vi "Check Next Step.vi"(8 "error in (no error)":errorcluster, 10 "Current Time":timestamp, 11 "Output Sequencer in":refnum<class "Output Sequencer.lvclass">) -> (0 "error out":errorcluster, 2 "Go to Next Step":bool, 3 "Output Sequencer out":refnum<class "Output Sequencer.lvclass">, 4 "Current Step End Timestamp":dbl)   [LabVIEW 2020, in "Output Sequencer.lvlib" / "Output Sequencer.lvclass"]
uses:
  Output Sequencer.lvclass
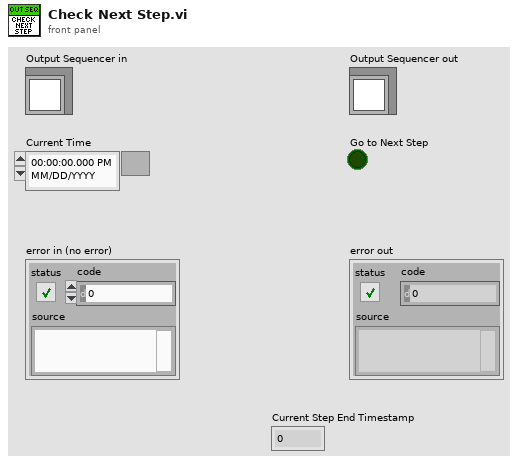
[diagram p1: front panel]
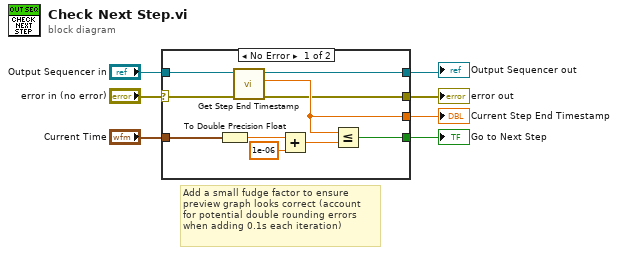
[diagram p0: block diagram]
diagram:
  # "Add a small fudge factor to ensure\npreview graph looks correct (account\nfor potential double rounding errors\nwhen adding 0.1s each iteration)"
  n1 = case shown="No Error" "error in (no error)" {
    selector: "error in (no error)" -> [w8 w18]
    tunnel: "Output Sequencer in" -> [w17 w19]
    tunnel: [w16 _] -> w6
    tunnel: [w15 _] -> w5
    tunnel: [w14 w18] -> w4
    tunnel: [w13 w19] -> w3
    tunnel: "Current Time" -> [w12 _]
    frame No Error {
      n2 = To Double Precision Float(number=w12) -> (double precision float=w10:dbl)
      n3 = call "Get Step End Timestamp.vi"("error in (no error)"=w8, "Output Sequencer in"=w17) -> ("error out"=w14:errorcluster, "Current Step End Timestamp"=w15:dbl, "Output Sequencer out"=w13:refnum<class "Output Sequencer.lvclass">)  [unwired: 7 in]
      n4 = Add(x=w10, y=1e-06) -> (x+y=w9:dbl)
      n5 = Less Or Equal?(x=w15, y=w9) -> (x <= y?=w16:bool)
    }
    frame Error {
    }
  }
  "Go to Next Step" <- w6
  "Current Step End Timestamp" <- w5
  "error out" <- w4
  "Output Sequencer out" <- w3
